vi "conf_tabla_P031.vi"(11 "Prueba07 out":refnum<class "Prueba031.lvclass">) -> (0 "cumplimiento":string[](array[string]), 1 "Tol -":string[](array[string]), 2 "Tol +":string[](array[string]), 3 "incertidumbre":string[](array[string]))   [LabVIEW 2019, in "Prueba031.lvclass"]
uses:
  Prueba031.lvclass
  Prueba031.lvclass/Prueba031.ctl
panel:
  out "Array 3":string[](array[string])
  out "Array 2":string[](array[string])
  out "Array":string[](array[string])
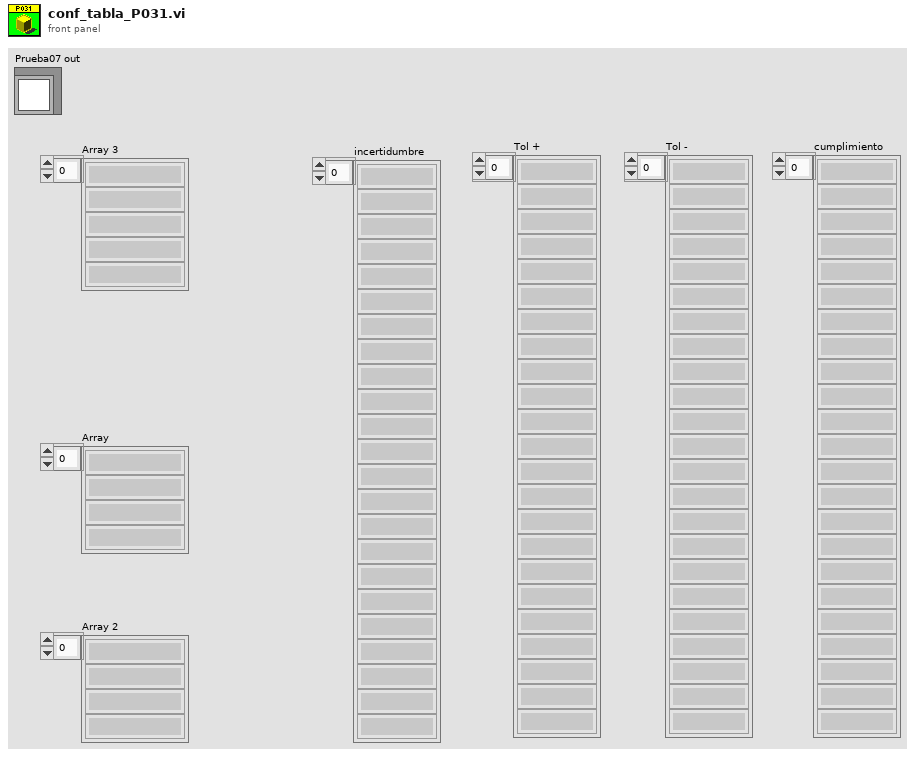
[diagram p1: front panel]
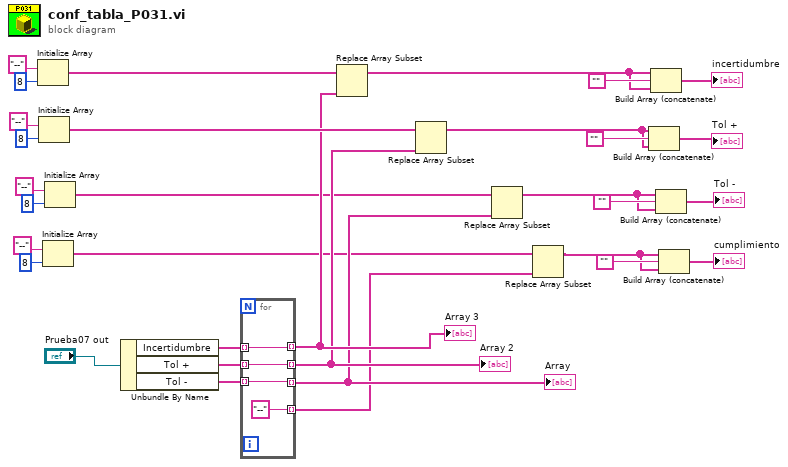
[diagram p0: block diagram]
diagram:
  n1 = Initialize Array("--" ("format string"), 8 ("dimension size")) -> (w25:string[])
  n2 = Initialize Array("--" ("format string"), 8 ("dimension size")) -> (w26:string[])
  n3 = Initialize Array("--" ("format string"), 8 ("dimension size")) -> (w5:string[])
  n4 = Initialize Array("--" ("format string"), 8 ("dimension size")) -> (w10:string[])
  n5 = Unbundle By Name("Prueba07 out") -> ("Incertidumbre"=w19:string[], "Tol +"=w18:string[], "Tol -"=w17:string[])
  n6 = for {
    tunnel: w19 -> [w36] mode=indexing
    tunnel: w18 -> [w35] mode=indexing
    tunnel: w17 -> [w34] mode=indexing
    tunnel: [w36] -> w14 mode=indexing
    tunnel: [w35] -> w13 mode=indexing
    tunnel: [w34] -> w8 mode=indexing
    tunnel: ["--" ("format string")] -> w1 mode=indexing
  }
  "Array" <- w8
  "Array 2" <- w13
  "Array 3" <- w14
  n7 = Replace Array Subset(array=w25, new element=w14) -> (w23:string[])  [unwired: 1 in]
  n8 = Replace Array Subset(array=w26, new element=w13) -> (w16:string[])  [unwired: 1 in]
  n9 = Replace Array Subset(array=w10, new element=w8) -> (w9:string[])  [unwired: 1 in]
  n10 = Replace Array Subset(array=w5, new element=w1) -> (w2:string[])  [unwired: 1 in]
  n11 = Build Array (concatenate)(w16, "", w16) -> (→"Tol +":string[])
  n12 = Build Array (concatenate)(w23, "", w23) -> (→"incertidumbre":string[])
  n13 = Build Array (concatenate)(w9, "", w9) -> (→"Tol -":string[])
  n14 = Build Array (concatenate)(w2, "", w2) -> (→"cumplimiento":string[])
